vi "Update Calibration Settings (Array).vi"(2 "Calibration Settings ducktype":T1(array[cluster]), 3 "Channel Settings in":T2[](array[typedef])) -> (0 "Channel Settings out":T2[](array[typedef]))   [LabVIEW 2021, in "Settings.lvlib"]
uses:
  Acquisition/Channel Settings.ctl
  Acquisition/IO Device.ctl
  Acquisition/Sensor Type.ctl
  Settings.lvlib
  Acquisition/Acquisition.lvlib
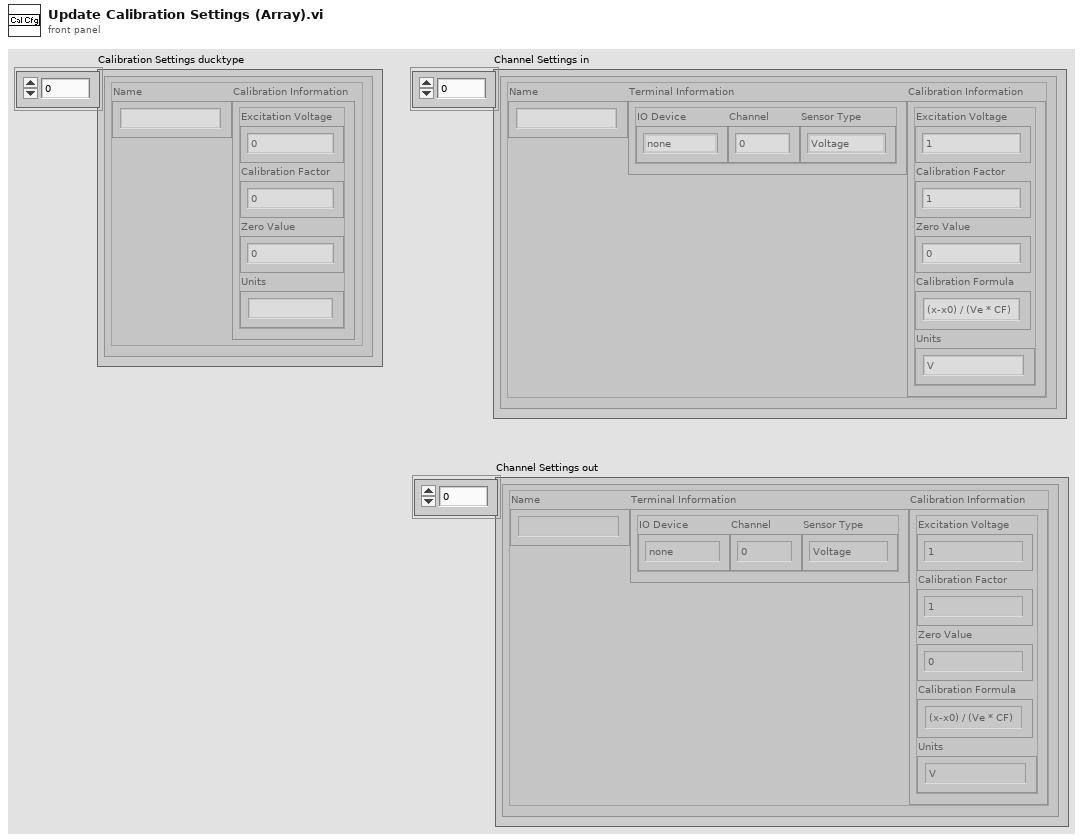
[diagram p1: front panel]
types:
  T1 = cluster{"Name":string, "Calibration Information":cluster{"Excitation Voltage":dbl, "Calibration Factor":dbl, "Zero Value":dbl, "Units":string}}[]
  T2 = typedef "Acquisition.lvlib/Channel Settings.ctl" = cluster{"Name":string, "Terminal Information":cluster{"IO Device":T3, "Channel":i32, "Sensor Type":T4}, "Calibration Information":cluster{"Excitation Voltage":dbl, "Calibration Factor":dbl, "Zero Value":dbl, "Calibration Formula":string, "Units":string}}
  T3 = typedef "Acquisition.lvlib/IO Device.ctl" = enum16{"none", "9219", "9401"}
  T4 = typedef "Acquisition.lvlib/Sensor Type.ctl" = enum16{"Voltage", "Load", "Pressure", "Encoder"}
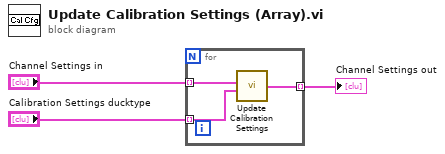
[diagram p0: block diagram]
diagram:
  n1 = for {
    tunnel: "Calibration Settings ducktype" -> [w5] mode=indexing
    tunnel: "Channel Settings in" -> [w6] mode=indexing
    tunnel: [w4] -> w1 mode=indexing
    n2 = call "Update Calibration Settings.vi"("Calibration Settings ducktype"=w5, "Channel Settings in"=w6) -> ("Channel Settings out"=w4:T2)  [unwired: 2 in]
  }
  "Channel Settings out" <- w1
